vi "Update.vi"(11 "服务器信息":T1={"host"="27.154.58.30", "user"="fb", "password"="std23506", "远端地址"="/微站/室外总磷总氮高压过滤无主板新电路板/一体化微型水质监测站.exe"}) -> ()   [LabVIEW 2016, in "update.lvlib"]
uses:
  update.lvlib
panel:
  out "滑动杆":dbl(slide) scale=0.0..100.0
  in  "取消按钮":bool
  out "last status string":string caption="最近状态字符串"
  out "command":string caption="命令"
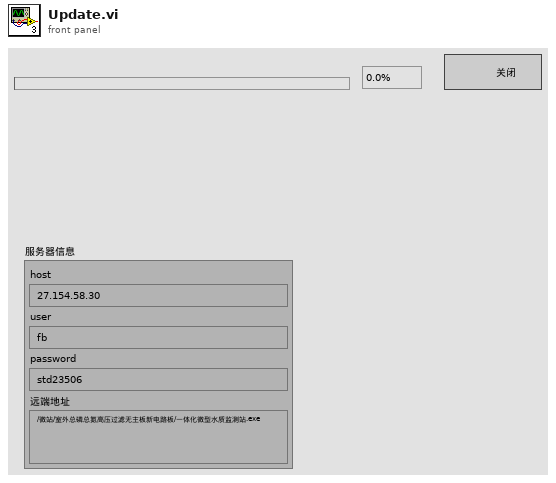
[diagram p1: front panel]
types:
  T1 = cluster{"host":string, "user":string, "password":string, "远端地址":string}
  T2 = cluster{"command":string, "last status string":string, "process":dbl}
  T3 = enum32{"Bad", "Idle", "Run top level", "Running"}
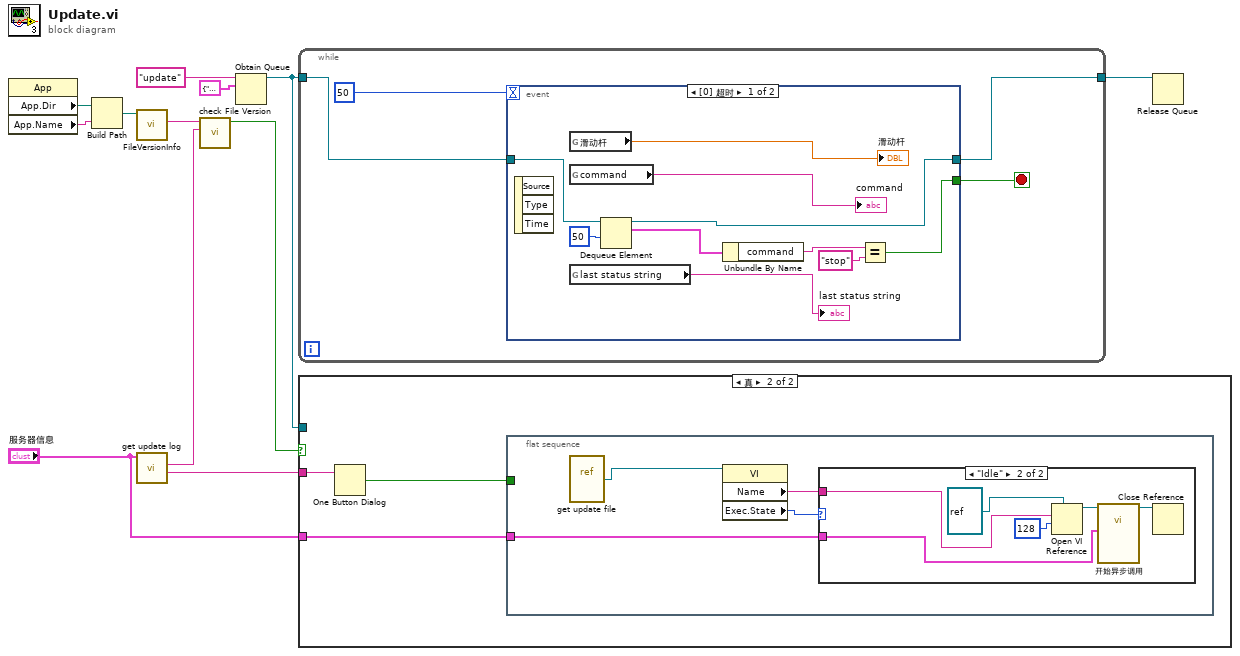
[diagram p0: block diagram]
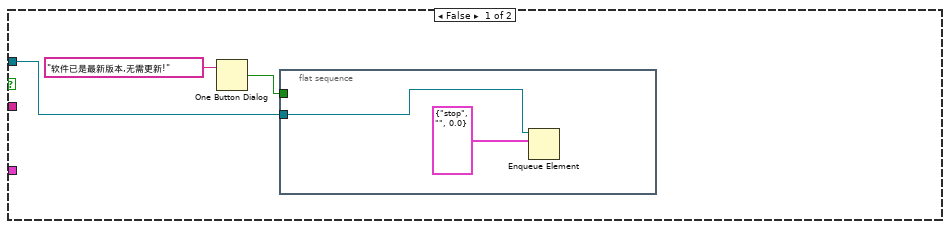
[diagram p2: hidden frame]
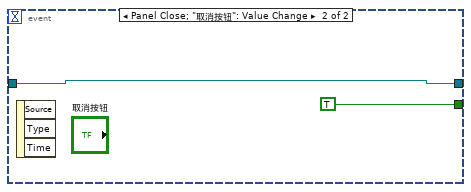
[diagram p4: hidden frame]
diagram:
  n1 = property class="App"() -> ("App.Dir"=w7:path, "App.Name"=w6:string)  [unwired: 2 in, 2 out]
  n2 = Build Path(base path=w7, name or relative path=w6) -> (appended path=w5:path)
  n3 = call <vilib>:"FileVersionInfo.vi"("Application Path in"=w5) -> ("File Version Info"=w4:string)  [unwired: 7 in, 3 out]
  n4 = call "get update log.vi"("服务器信息"="服务器信息") -> ("部分更新日志"=w1:string, "remote File Version"=w8:string)  [unwired: 7 in, 2 out]
  n5 = call "check File Version.vi"("remote File Version Info"=w8, "Local File Version Info"=w4) -> ("new?"=w3:bool)  [unwired: 9 in]
  n6 = Obtain Queue(name (unnamed)="update" ("名称（未命名）"), element data type=T2 {"command"="", "last status string"="", "process"=0.0}) -> (queue out=w2:refnum<queue>)  [unwired: 3 in, 2 out]
  n7 = while {
    tunnel: w2 -> [w14]
    tunnel: [w13] -> w11
    stop <- w15 stop-if-true
    n8 = event shown="[0] 超时" {
      selector: _ -> [_ _]
      dyn-events: _ -> [_ _]
      timeout: 50 -> [_ _]
      tunnel: [w21 TRUE] -> w15
      tunnel: w14 -> [w26 w27]
      tunnel: [w24 w27] -> w13
      event Timeout {
        n9 = event-data() -> ()  [unwired: 1 in, 3 out]
        n10 = global read "更新全局变量.vi" "滑动杆"() -> (→"滑动杆":dbl)
        n11 = global read "更新全局变量.vi" "command"() -> (→"command":string)
        n12 = global read "更新全局变量.vi" "last status string"() -> (→"last status string":string)
        n13 = Dequeue Element(queue=w26, timeout in ms (-1)=50 ("超时毫秒(-1)")) -> (queue out=w24:refnum<queue>, element=w25:T2)  [unwired: 1 in, 2 out]
        n14 = Unbundle By Name(w25) -> ("command"=w23:string)
        n15 = Equal?(x=w23, y="stop") -> (x = y?=w21:bool)
      }
      event Panel Close; "取消按钮": Value Change {
        n16 = event-data() -> ()  [unwired: 1 in, 3 out]
      }
    }
  }
  n17 = case shown="真" w3 {
    tunnel: "服务器信息" -> [_ w36]
    tunnel: w1 -> [_ w35]
    tunnel: w2 -> [w30 _]
    frame False {
      n18 = One Button Dialog(message="软件已是最新版本,无需更新!" ("消息")) -> (true=w29:bool)  [unwired: 1 in]
      n19 = flat-sequence {
        tunnel: w30 -> [w33]
        tunnel: w29 -> [_]
        frame #0 {
          n20 = Enqueue Element(queue=w33, element=T2 {"command"="stop", "last status string"="", "process"=0.0} ("元素")) -> ()  [unwired: 2 in, 3 out]
        }
      }
    }
    frame True {
      n21 = One Button Dialog(message=w35) -> (true=w34:bool)  [unwired: 1 in]
      n22 = flat-sequence {
        tunnel: w36 -> [w37]
        tunnel: w34 -> [_]
        frame #0 {
          n23 = vi-ref "get update file.vi"() -> (w40:refnum<vi>)
          n24 = property class="VI"(reference=w40) -> ("Name"=w39:string, "Exec.State"=w38:T3)  [unwired: 1 in, 2 out]
          n25 = case shown="\"Idle\"" w38 {
            tunnel: w39 -> [_ w46]
            tunnel: w37 -> [_ w41]
            frame "Bad", Default {
            }
            frame "Idle" {
              n26 = Open VI Reference(type specifier VI Refnum (for type only)=refnum<vi> refnum, vi path=w46, options=128 ("选项")) -> (vi reference=w43:refnum<vi>)  [unwired: 3 in, 1 out]
              n27 = call-by-ref "开始异步调用"(reference=w43, "服务器信息"=w41) -> (reference out=w44:refnum<vi>)  [unwired: 12 in, 1 out]
              n28 = Close Reference(reference=w44) -> ()  [unwired: 1 in, 1 out]
            }
          }
        }
      }
    }
  }
  n29 = Release Queue(queue=w11) -> ()  [unwired: 2 in, 3 out]
